vi "programa 9.vi"() -> ()   [LabVIEW 2011]
panel:
  in  "on/off Prg":bool
  out "TempMinima 2":dbl
  out "TempMaxima":dbl
  out "TempPromedio":dbl
  in  "on/off A/C":bool
  out "A/C on":bool
  in  "TempDeseada":dbl
  out "Temperatura":i32(slide) scale=0.0..50.0
  # "El programa simula el funcionamiento de un A/C\ndonde se ingresa la temperatura deseada y cada\nvez que la temperatura deseada sea mayor a \ntemperatura no se enciende el compresor del\nA/C, pero cuando este sea menor se enciende  el compresor\npero esto solo puede ocurrir siempre que el A/C este \nencendido, el programa termina solo cuando decidimos\nnosotros terminar."
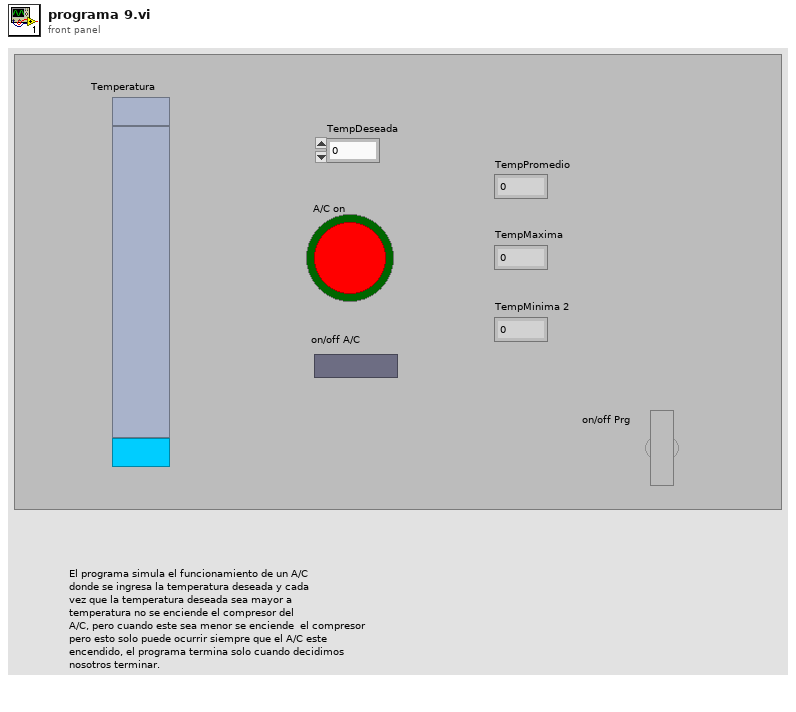
[diagram p1: front panel]
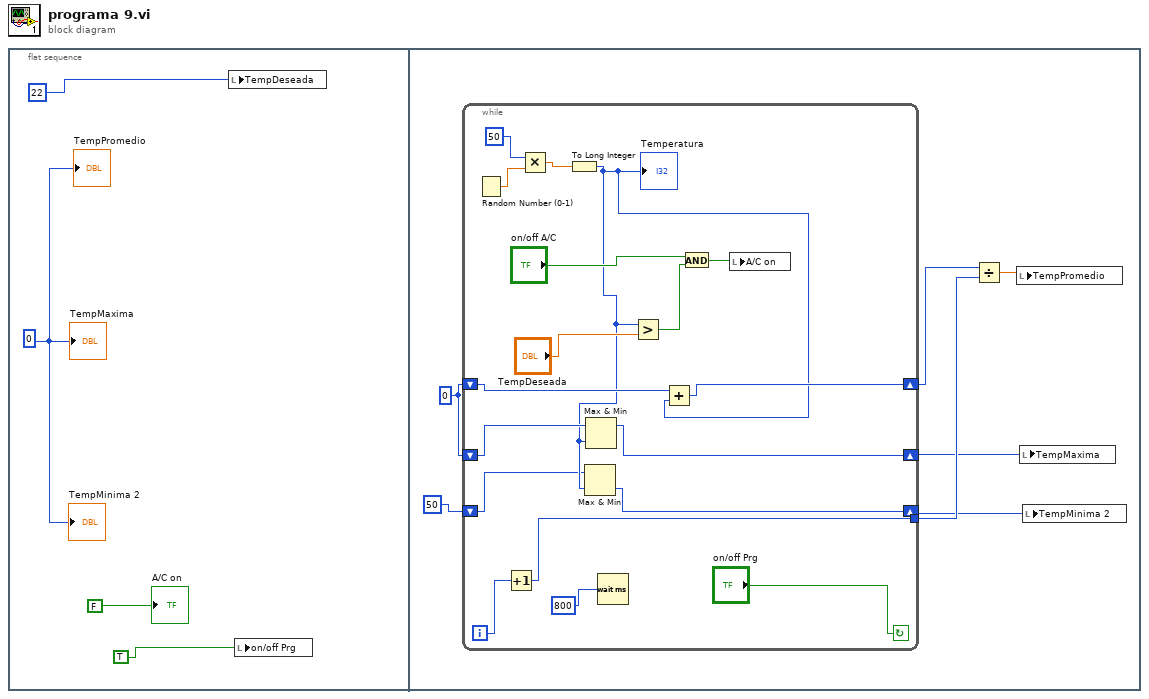
[diagram p0: block diagram]
diagram:
  n1 = flat-sequence {
    frame #0 {
      w4 = 0
      n2 = local write "TempDeseada"(22) -> ()
      n3 = local write "on/off Prg"(TRUE) -> ()
      "A/C on" <- FALSE
      "TempPromedio" <- w4
      "TempMaxima" <- w4
      "TempMinima 2" <- w4
    }
    frame #1 {
      w8 = 0
      n4 = while {
        tunnel: [w19] -> w10
        shift-right: [w17] -> w9
        shift-left: w8 -> [w18]
        shift-right: [w13] -> w6
        shift-left: w8 -> [w16]
        shift-right: [w12] -> w7
        shift-left: 50 -> [w14]
        i -> [w20]
        stop <- "on/off Prg" continue-if-true
        n5 = Random Number (0-1)() -> (number: 0 to 1=w27:dbl)
        n6 = Increment(x=w20) -> (x+1=w19:i32)
        n7 = Multiply(x=50, y=w27) -> (x*y=w26:dbl)
        n8 = To Long Integer(number=w26) -> (32bit integer=w15:i32)
        "Temperatura" <- w15
        n9 = Max & Min(x=w14, y=w15) -> (min(x,y)=w12:i32)  [unwired: 1 out]
        n10 = Max & Min(x=w16, y=w15) -> (max(x,y)=w13:i32)  [unwired: 1 out]
        n11 = Wait (ms)(milliseconds to wait=800) -> ()  [unwired: 1 out]
        n12 = Greater?(x=w15, y="TempDeseada") -> (0:w23:bool)
        n13 = Add(x=w18, y=w15) -> (x+y=w17:i32)
        n14 = And(x="on/off A/C", y=w23) -> (x .and. y?=w21:bool)
        n15 = local write "A/C on"(w21) -> ()
      }
      n16 = Divide(x=w9, y=w10) -> (x/y=w11:dbl)
      n17 = local write "TempPromedio"(w11) -> ()
      n18 = local write "TempMaxima"(w6) -> ()
      n19 = local write "TempMinima 2"(w7) -> ()
    }
  }
